vi "Test Filesaving Vi.vi"() -> ()   [LabVIEW 2018]
panel:
  out "Sine with Uniform Noise":dbl=0.05394995810837566
  in  "stop":bool
  out "tdms error":errorcluster
  out "tdms file":refnum<k34>
  in  "Measurement number":i32
  in  "Filename (Meas. Description)":string="Power_80C"
  out "Instrument":string="Spectrometer"
  in  "Folder (Project)":string="VAPORTUBE\\Temp Dependence"
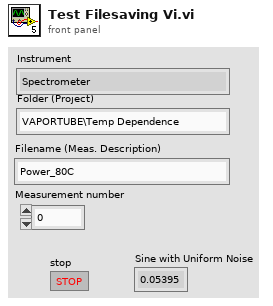
[diagram p1: front panel]
types:
  T1 = enum16{"Left Button", "Center Button", "Right Button", "Window Close"}
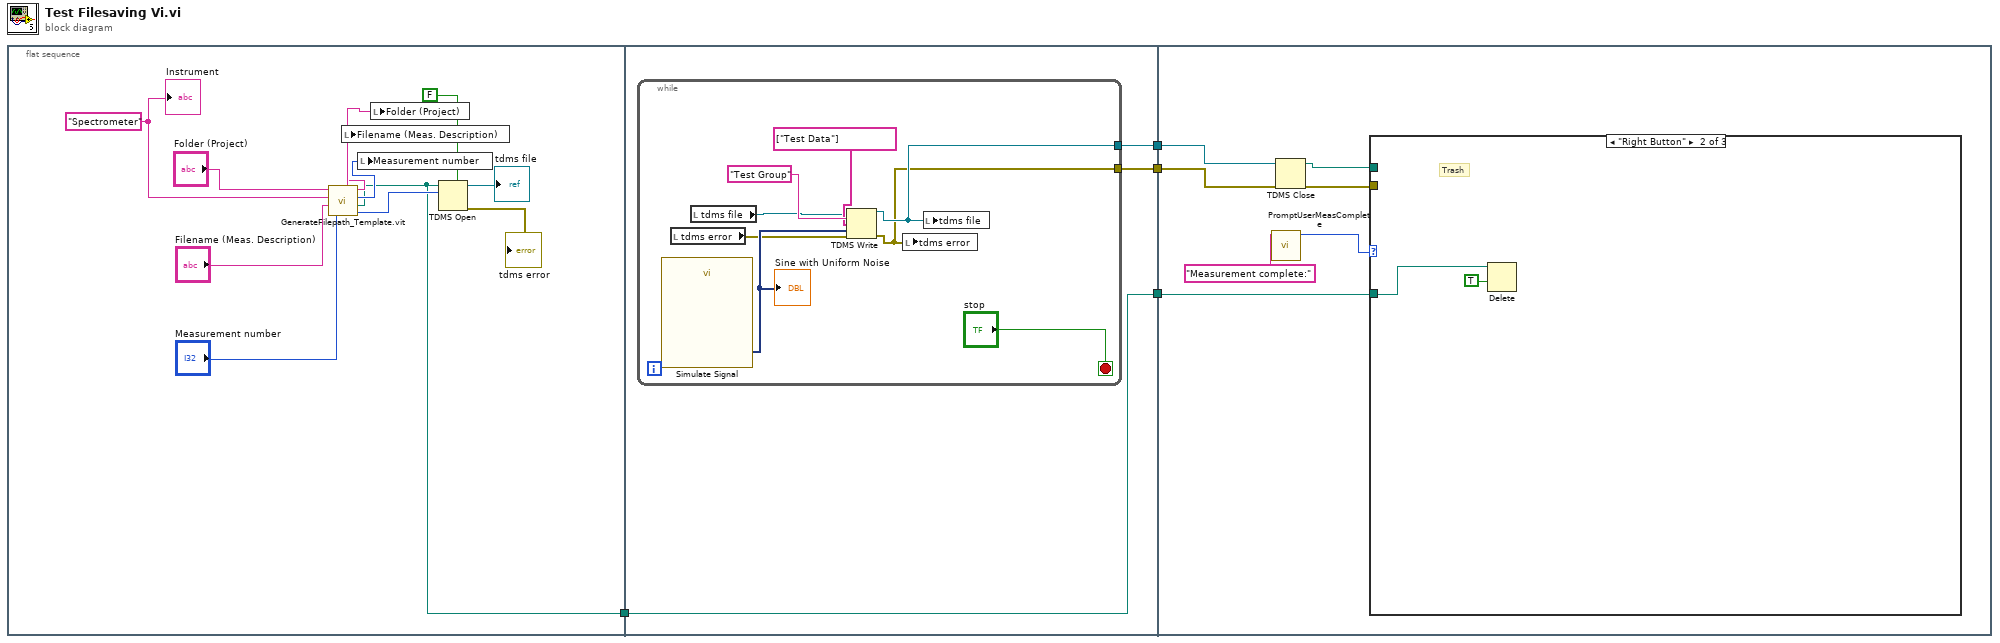
[diagram p0: block diagram]
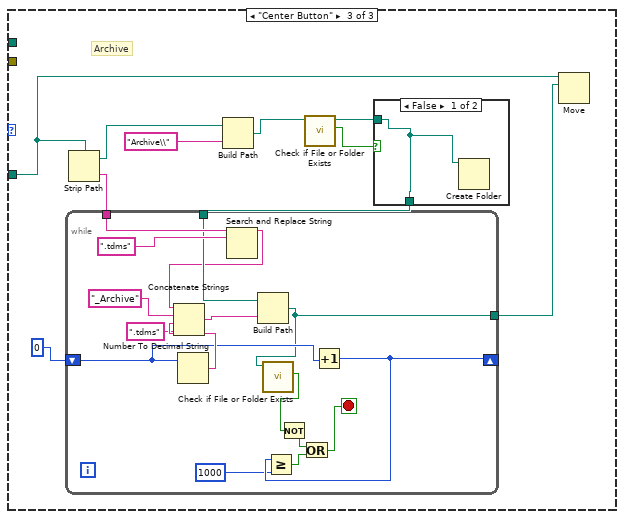
[diagram p3: hidden frame]
diagram:
  n1 = flat-sequence {
    tunnel: [w6] -> w1
    tunnel: [w19] -> w4
    tunnel: [w18] -> w3
    tunnel: [w17] -> w2
    tunnel: w1 -> [w17]
    tunnel: w4 -> [w32]
    tunnel: w3 -> [w31]
    tunnel: w2 -> [w33]
    frame #0 {
      w9 = "Spectrometer" ("Instrument")
      n2 = call "GenerateFilepath_Template.vit"("Project"="Folder (Project)", "Instrument"=w9, "Meas. Description"="Filename (Meas. Description)", "Measurement number"="Measurement number") -> ("Project Out"=w16:string, "Meas. Description Out"=w15:string, "Measurement number Out"=w14:i32, "File Path Out"=w6:path, "File Action"=w13:i32)
      n3 = local write "Filename (Meas. Description)"(w15) -> ()
      n4 = local write "Measurement number"(w14) -> ()
      n5 = local write "Folder (Project)"(w16) -> ()
      n6 = TDMS Open(5:FALSE ("create index file? (T)"), 10:w13, 11:w6) -> (0:→"tdms error":errorcluster, 3:→"tdms file":refnum<k34>)  [unwired: 4 in]
      "Instrument" <- w9
    }
    frame #1 {
      n7 = while {
        tunnel: [w21] -> w19
        tunnel: [w20] -> w18
        stop <- "stop" stop-if-true
        n8 = call "Simulate Signal"() -> ("Sine with Uniform Noise"=w24:dynamicdata)  [unwired: 14 in, 1 out]
        "Sine with Uniform Noise" <- w24
        n9 = local read "tdms error"() -> (w23:errorcluster)
        n10 = local read "tdms file"() -> (w25:refnum<k34>)
        n11 = TDMS Write(0:w25, 5:"Test Group" ("group name in (Untitled)"), 7:string[] ["Test Data"] ("channel name(s) in (Untitled)"), 9:w24, 11:w23) -> (4:w21:refnum<k34>, 15:w20:errorcluster)  [unwired: 1 in, 2 out]
        n12 = local write "tdms error"(w20) -> ()
        n13 = local write "tdms file"(w21) -> ()
      }
    }
    frame #2 {
      n14 = call "PromptUserMeasComplete.vi"("message"="Measurement complete:") -> ("Which Button?"=w34:T1)  [unwired: 10 in]
      n15 = TDMS Close(8:w31, 11:w32) -> (0:w29:errorcluster, 3:w30:path)
      n16 = case shown="\"Right Button\"" w34 {
        tunnel: w33 -> [_ w36 w46]
        tunnel: w30 -> [_ _ _]
        tunnel: w29 -> [_ _ _]
        frame "Left Button", Default {
        }
        frame "Right Button" {
          # "Trash"
          n17 = Delete(path (use dialog)=w36, confirm (F)=TRUE) -> ()  [unwired: 3 in, 3 out]
        }
        frame "Center Button" {
          # "Archive"
          n18 = Strip Path(path=w46) -> (stripped path=w45:path, name=w43:string)
          n19 = Build Path(base path=w45, name or relative path="Archive\\") -> (appended path=w40:path)
          n20 = call <vilib>:"Check if File or Folder Exists.vi"("path"=w40) -> ("file or folder exists?"=w39:bool, "dup path"=w38:path)  [unwired: 8 in, 1 out]
          n21 = case shown="False" w39 {
            tunnel: w38 -> [w47 w48]
            tunnel: [w47 w48] -> w37
            frame False {
              n22 = Create Folder(path (use dialog)=w47) -> ()  [unwired: 2 in, 3 out]
            }
            frame True {
            }
          }
          n23 = while {
            tunnel: w43 -> [w64]
            tunnel: w37 -> [w62]
            shift-right: [w50] -> _
            shift-left: 0 -> [w56]
            tunnel: [w52] -> w41
            stop <- w53 stop-if-true
            n24 = Number To Decimal String(number=w56) -> (decimal integer string=w60:string)  [unwired: 1 in]
            n25 = Search and Replace String(input string=w64, search string=".tdms") -> (result string=w51:string)  [unwired: 6 in, 3 out]
            n26 = Concatenate Strings(w51, "_Archive" ("replace string (\"\")"), w60, ".tdms" ("string")) -> (w58:string)
            n27 = Build Path(base path=w62, name or relative path=w58) -> (appended path=w52:path)
            n28 = call <vilib>:"Check if File or Folder Exists.vi"("path"=w52) -> ("file or folder exists?"=w57:bool)  [unwired: 8 in, 2 out]
            n29 = Not(x=w57) -> (.not. x?=w55:bool)
            n30 = Increment(x=w56) -> (x+1=w50:i32)
            n31 = Greater Or Equal?(x=w50, y=1000) -> (x >= y?=w54:bool)
            n32 = Or(x=w55, y=w54) -> (x .or. y?=w53:bool)
          }
          n33 = Move(source path=w46, 10:w41) -> ()  [unwired: 3 in, 3 out]
        }
      }
    }
  }
